vi "1.2.1.2-Generic ReadWrite.vi"(5 "RS232-1\\Port1 Read Timeout":bool=TRUE, 6 "2.2 Where Control":T1, 7 "RS232-1\\Port1 Write Timeout":bool=TRUE) -> (1 "RS232-1\\Port1 Read Case":bool, 2 "2.2 Where Indicator":T2, 3 "RS232-1\\Port1 Write Case":bool)   [LabVIEW 2011]
uses:
  2-Low Neurons/2.2-Where Indicator.ctl
  2-Low Neurons/2.2-Where Control.ctl
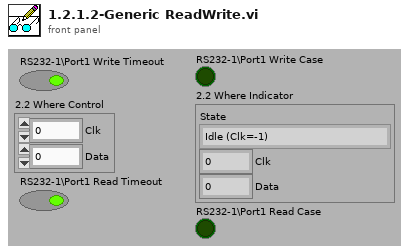
[diagram p1: front panel]
types:
  T1 = typedef "2.2-Where Control.ctl" = cluster{"Clk":i8, "Data":u8}
  T2 = typedef "2.2-Where Indicator.ctl" = cluster{"State":enum8{"Idle (Clk=-1)", "Sending(Clk*==Clk+1?Clk=Clk*:;)", "Receiving(Clk*==Clk?Clk++:;)"}, "Clk":i8, "Data":u8}
  T3 = enum8{"Idle (Clk=-1)", "Sending(Clk*==Clk+1?Clk=Clk*:;)", "Receiving(Clk*==Clk?Clk++:;)"}
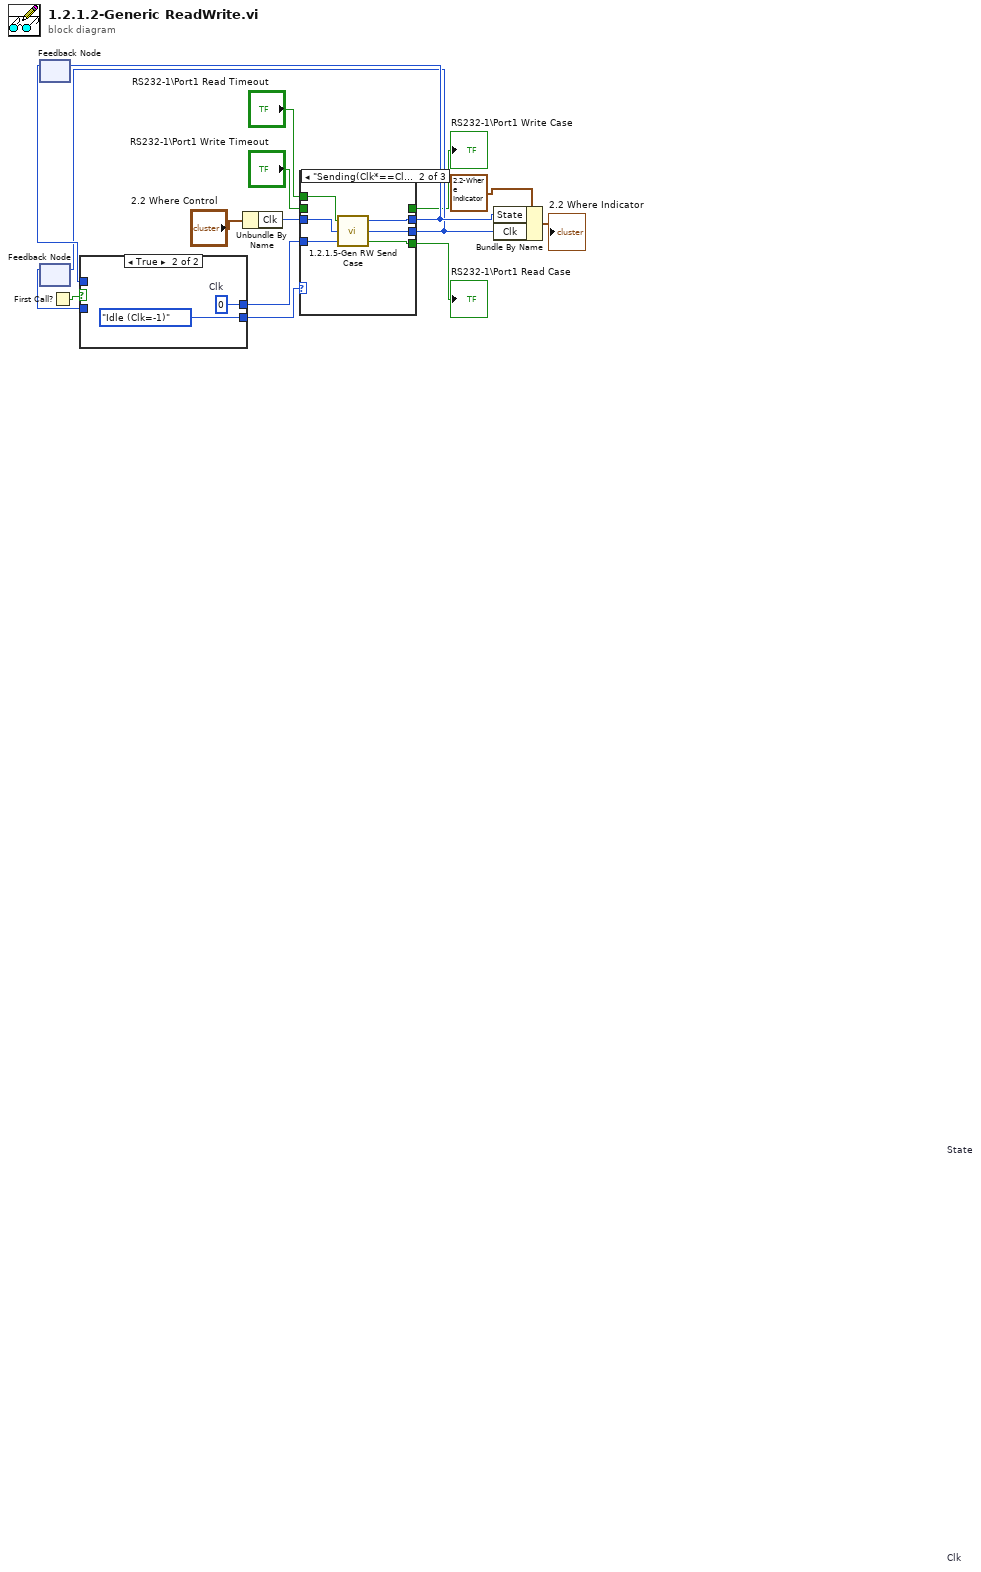
[diagram p0: block diagram]
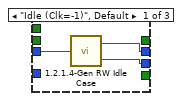
[diagram p3: hidden frame]
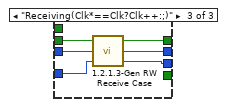
[diagram p4: hidden frame]
diagram:
  n1 = feedback #1 "State"() -> (w10:T3)  [unwired: 1 in]
  n2 = feedback #2 "Clk"() -> (w7:i8)  [unwired: 1 in]
  n3 = First Call?() -> (First Call?: T/F=w11:bool)
  n4 = case shown="True" w11 {
    tunnel: [w17 T3."Idle (Clk=-1)" ("State")] -> w9
    tunnel: w10 -> [w17 _]
    tunnel: [w16 w18] -> w8
    tunnel: w7 -> [w16 _]
    frame False {
    }
    frame True {
      w18 = i8 0  # Clk
    }
  }
  n5 = Unbundle By Name("2.2 Where Control") -> ("Clk"=w12:i8)
  n6 = case shown="\"Sending(Clk*==Clk+1?Clk=Clk*:;)\"" w9 {
    tunnel: w12 -> [w22 w26 w34]
    tunnel: [w21 w28 w29] -> w6
    tunnel: [w20 w25 w30] -> w5
    tunnel: w8 -> [_ w27 w33]
    tunnel: [_ _ w31] -> w4
    tunnel: "RS232-1\\Port1 Read Timeout" -> [_ w23 _]
    tunnel: "RS232-1\\Port1 Write Timeout" -> [_ _ w32]
    tunnel: [_ w24 _] -> w1
    frame "Idle (Clk=-1)", Default {
      n7 = call "1.2.1.4-Gen RW Idle Case.vi"("Clk"=w22) -> ("Clk=-1;"=w20:i8, "State"=w21:T3)
    }
    frame "Sending(Clk*==Clk+1?Clk=Clk*:;)" {
      n8 = call "1.2.1.5-Gen RW Send Case.vi"("Local Clock: Clk"=w27, "Foreign Clock: Clk*"=w26, "RS232-1\\Port1 Read Timeout"=w23) -> ("RS232-1\\Port1 Read"=w24:bool, "New Local Clock: Clk"=w25:i8, "State"=w28:T3)
    }
    frame "Receiving(Clk*==Clk?Clk++:;)" {
      n9 = call "1.2.1.3-Gen RW Receive Case.vi"("Local Clock: Clk"=w33, "Foreign Clock: Clk*"=w34, "RS232-1\\Port1 Write Timeout"=w32) -> ("New Local Clock: Clk"=w30:i8, "State"=w29:T3, "RS232-1\\Port1 Write"=w31:bool)
    }
  }
  "RS232-1\\Port1 Write Case" <- w4
  "RS232-1\\Port1 Read Case" <- w1
  n10 = feedback-in #1(w6) -> ()
  n11 = feedback-in #2(w5) -> ()
  n12 = Bundle By Name(cluster=T2 {"State"=enum."Sending(Clk*==Clk+1?Clk=Clk*:;)", "Clk"=0, "Data"=0} ("2.2 Where Indicator"), "State"=w6, "Clk"=w5) -> (→"2.2 Where Indicator":T2)
